vi "RelDisplay.vi"(7 "Boolean":bool, 11 "error in (no error)":errorcluster) -> (6 "Answer":string, 8 "Boolean":bool, 15 "error out":errorcluster)   [LabVIEW 2014, in "FH 55.lvlib"]
doc: "Dieses VI gibt nur den aktuellen Temperaturwert zurück wenn Celsius oder Fahrenheit übergeben wird.\n\nThis VI returns only the current temperature where Celsius and Fahrenheit is inputted."
uses:
  FH 55.lvlib
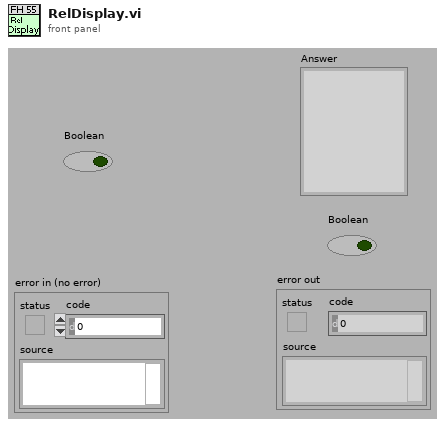
[diagram p1: front panel]
types:
  T1 = typedef "FH 55.lvlib/Value_String.ctl" = cluster{"Numeric":dbl, "String":string}
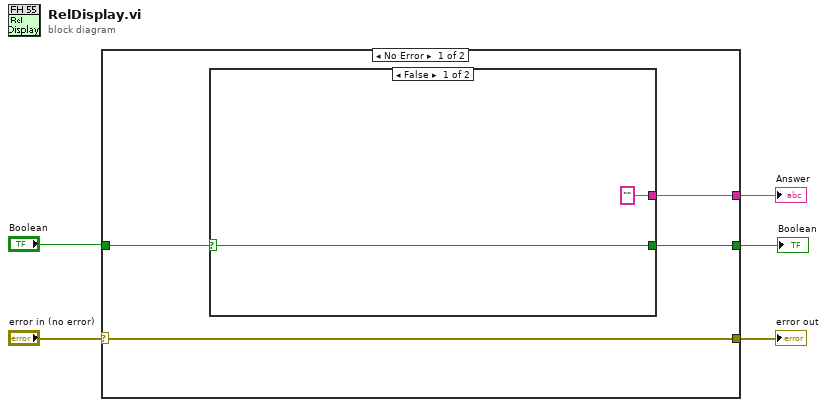
[diagram p0: block diagram]
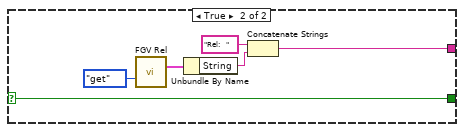
[diagram p2: hidden frame]
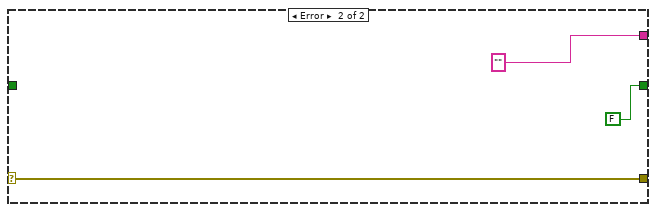
[diagram p3: hidden frame]
diagram:
  n1 = case shown="No Error" "error in (no error)" {
    selector: "error in (no error)" -> [w6 w20]
    tunnel: [w8 "" ("Answer")] -> w5
    tunnel: "Boolean" -> [w9 _]
    tunnel: [w6 w20] -> w3
    tunnel: [w7 FALSE] -> w1
    frame No Error {
      n2 = case shown="False" w9 {
        selector: w9 -> [w10 w14]
        tunnel: ["" w15] -> w8
        tunnel: [w10 w14] -> w7
        frame False {
        }
        frame True {
          n3 = call "FGV Rel.vi"("action"=enum16{"set", "get"}."get") -> ("Extrem_Value"=w13:T1)  [unwired: 13 in, 1 out]
          n4 = Unbundle By Name(w13) -> ("String"=w12:string)
          n5 = Concatenate Strings("Rel:   " ("string"), w12) -> (w15:string)
        }
      }
    }
    frame Error {
    }
  }
  "Answer" <- w5
  "error out" <- w3
  "Boolean" <- w1
